vi "convert_and_assert.vi"(8 "error in (no error)":errorcluster, 9 "Config String (\"\")":string, 10 "Config String (\"\") 2":string, 11 "Label":string) -> (0 "error out":errorcluster, 2 "converted toml out":string)   [LabVIEW 2020]
uses:
  configuration-data/configuration-data.lvclass/configuration-data.ctl
  configuration-data/configuration.get.vi
  configuration-data/configuration.set.vi
  <vilib>/addons/_JKI.lib/_jki_lib_configuration_file.llb/Open Config String__jki_lib_configuration_file.vi
  <vilib>/Utility/config.llb/Get Section Names.vi
  <vilib>/Utility/config.llb/Get Key Names.vi
  <vilib>/Utility/config.llb/Read Key.vi
  <vilib>/Utility/config.llb/Read Key (String).vi
  configuration-data/datatype_conversion.vi
  <vilib>/Utility/config.llb/Close Config Data.vi
  configuration-data/configuration-data.lvclass
  <vilib>/addons/_JKI Toolkits/Caraya/classes/Assert/Assert Equal Value and Type_Variant.vi
  <vilib>/addons/_JKI Toolkits/Caraya/classes/Assert/Assert.lvclass
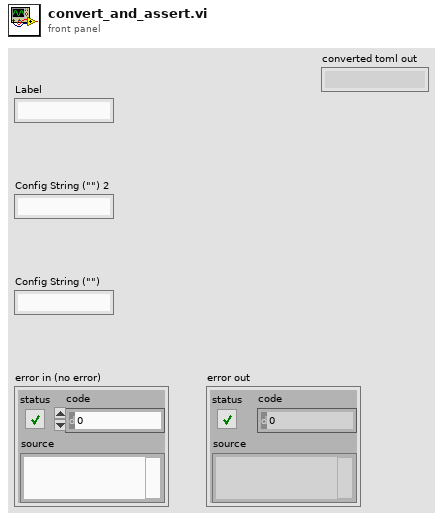
[diagram p1: front panel]
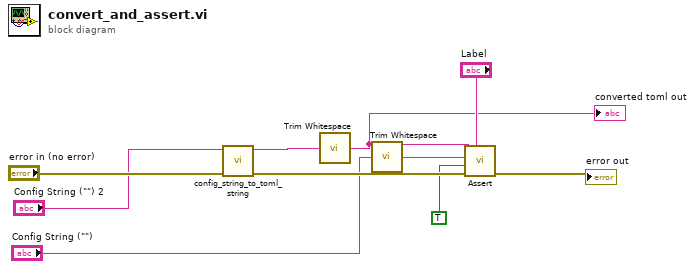
[diagram p0: block diagram]
diagram:
  n1 = call "config_string_to_toml_string.vi"("error in (no error)"="error in (no error)", "Config String (\"\") in"="Config String (\"\") 2") -> ("error out"=w10:errorcluster, "toml"=w4:string)  [unwired: 8 in]
  n2 = call <vilib>:"Trim Whitespace.vi"("string"=w4) -> ("trimmed string"=w1:string)  [unwired: 1 in]
  "converted toml out" <- w1
  n3 = call <vilib>:"Trim Whitespace.vi"("string"="Config String (\"\")") -> ("trimmed string"=w7:string)  [unwired: 1 in]
  n4 = call-poly <vilib>:"Assert.vi"("Label"="Label", "error in (no error)"=w10, "Register with caller test (F)"=TRUE, "Y"=w7, "X"=w1) -> ("error out"=→"error out":errorcluster)  [unwired: 6 in]
